vi "TimeSeriesSplit.vi"(6 "Groups":string[][](array[string]), 8 "error in (no error)":errorcluster caption="entrée d'erreur (pas d'erreur)", 9 "y":string[][](array[string]), 10 "X":string[][](array[string]), 11 "TimeSeriesSplit":cluster{"n_splits":i32, "max_train_size":string}={"n_splits"=5, "max_train_size"="None"}) -> (0 "error out":errorcluster caption="sortie d'erreur", 3 "Split":T1(array[cluster]))   [LabVIEW 2020]
doc: "Time Series cross-validator\n\nProvides train/test indices to split time series data samples that are observed at fixed time intervals, in train/test sets. In each split, test indices must be higher than before, and thus shuffling in cross validator is inappropriate.\n\nThis cross-validation object is a variation of KFold. In the kth split, it returns first k folds as train set and the (k+1)th fold as test set.\n\nNote that unlike standard cross-validation methods, successive training sets are supersets of those that come before them.\n\n\nParameters :\n\n- n_splits : int, default=5\nNumber of splits. Must be at least 2.\n\n- max_train_size : int, default=None\nMaximum size for a single training set.\n\n\n\nMethods : Split\n\n\nGenerate indices to split data into training and test set.\n\nParameters : \n\n- X : array-like of shape (n_samples, n_features)\nTraining data, where n_samples is the number of samples and n_features is the number of features.\n\n- y : array-like of shape (n_samples,)\nAlways ignored, exists for compatibility.\n\n- groups : array-like of shape (n_samples,)\nAlways ignored, exists for compatibility.\n\nYields :\n\n- train : ndarray\nThe training set indices for that split.\n\n- test : ndarray\nThe testing set indices for that split."
uses:
  TimeSeriesSplit.lvclass
panel:
  out "TimeSeriesSplit.lvclass":refnum<class "TimeSeriesSplit.lvclass">
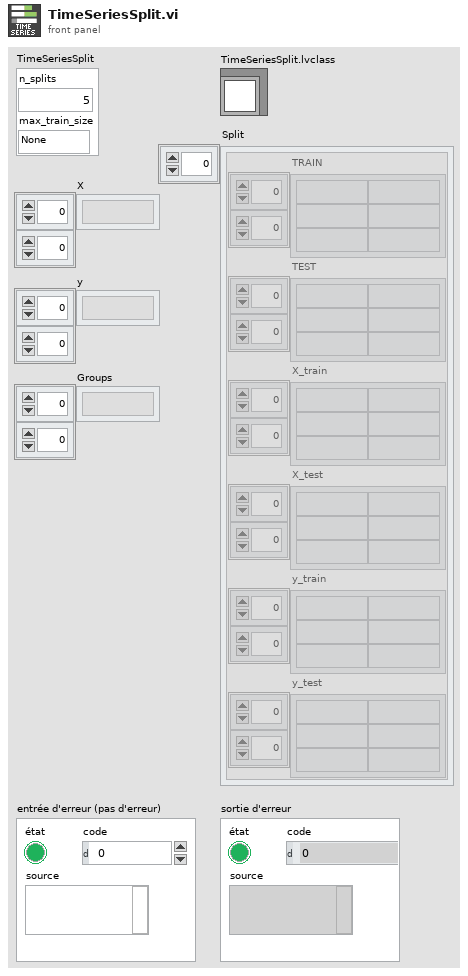
[diagram p1: front panel]
types:
  T1 = cluster{"TRAIN":string[][], "TEST":string[][], "X_train":string[][], "X_test":string[][], "y_train":string[][], "y_test":string[][]}[]
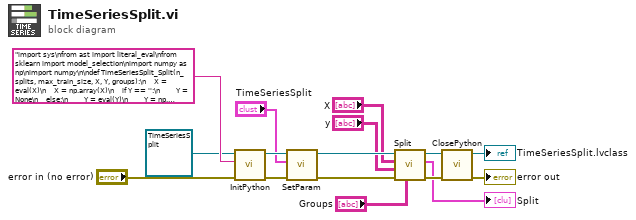
[diagram p0: block diagram]
diagram:
  n1 = call-dynamic "InitPython.vi"("error in (no error)"="error in (no error)", "Python Instruction"="import sys\nfrom ast import literal_eval\nfrom sklearn import model_selection\nimport numpy as np\nimport numpy\n\ndef TimeSeriesSplit_Split(n_splits, max_train_size, X, Y, groups):\n    X = eval(X)\n    X = np.array(X)\n    if Y == '':\n        Y = None\n    else:\n        Y = eval(Y)\n        Y = np.array(Y)\n    if groups == '':\n        groups = None\n    else:\n        groups = eval(groups)\n        groups = np.array(groups)\n    if max_train_size == 'None':\n        max_train_size = None\n    else:\n         max_train_size = eval(max_train_size)\n    list_return = []\n    try:\n        for train_index, test_index in model_selection.TimeSeriesSplit(n_splits, max_train_size).split(X, Y, groups):\n            list_return = list_return +[\"TRAIN:\", train_index.tolist(), \"TEST:\", test_index.tolist()]\n            X_train, X_test = X[train_index].tolist(), X[test_index].tolist()\n            y_train, y_test = Y[train_index].tolist(), Y[test_index].tolist()\n            list_return = list_return +[\"X_train:\", X_train, \"X_test:\", X_test, \"y_train:\", y_train, \"y_test:\", y_test]\n        return str(list_return)\n    except:\n        erreur = sys.exc_info()\n        typerr = u\"%s\" % (erreur[0])\n        typerr = typerr[typerr.find(\"'\")+1:typerr.rfind(\"'\")]\n        msgerr = u\"%s\" % (erreur[1])\n        message = str('/!\\\\ {0} : {1}'. format(typerr,msgerr))\n        return message", "Scikit-learn en entrée"=refnum<class "TimeSeriesSplit.lvclass"> refnum ("TimeSeriesSplit.lvclass")) -> ("error out"=w14:errorcluster, "Scikit-learn en sortie"=w13:refnum<class "TimeSeriesSplit.lvclass">)  [unwired: 7 in]
  n2 = call-dynamic "SetParam.vi"("error in (no error)"=w14, "TimeSeriesSplit"="TimeSeriesSplit", "TimeSeriesSplit.lvclass"=w13) -> ("error out"=w10:errorcluster, "TimeSeriesSplit.lvclass"=w9:refnum<class "TimeSeriesSplit.lvclass">)  [unwired: 7 in]
  n3 = call-dynamic "Split.vi"("Groups"="Groups", "error in (no error)"=w10, "y"="y", "X"="X", "TimeSeriesSplit.lvclass"=w9) -> ("error out"=w8:errorcluster, "Split"=→"Split":T1, "TimeSeriesSplit.lvclass"=w7:refnum<class "TimeSeriesSplit.lvclass">)  [unwired: 4 in]
  n4 = call-dynamic "ClosePython.vi"("error in (no error)"=w8, "Scikit-learn en entrée"=w7) -> ("error out"=→"error out":errorcluster, "Scikit-learn en sortie"=→"TimeSeriesSplit.lvclass":refnum<class "TimeSeriesSplit.lvclass">)  [unwired: 8 in]
